vi "Unreserve(Session).vi"(8 "error in (no error)":errorcluster, 9 "InstrumentHandle_port in":u32[](array[numeric]), 10 "InstrumentHandle_board in":u32[](array[numeric])) -> (0 "error out":errorcluster)   [LabVIEW 2020, in "AIM664LV.lvlib"]
uses:
  AIM664LV.lvlib
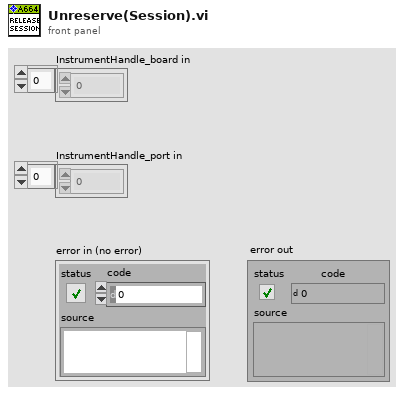
[diagram p1: front panel]
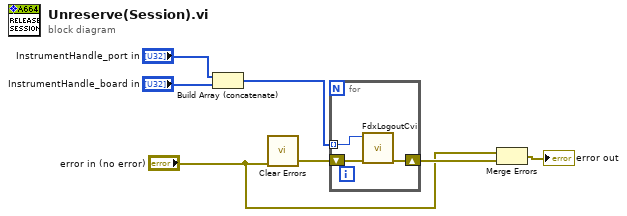
[diagram p0: block diagram]
diagram:
  n1 = Build Array (concatenate)("InstrumentHandle_port in", "InstrumentHandle_board in") -> (w1:u32[])
  n2 = call <vilib>:"Clear Errors.vi"("error in (no error)"="error in (no error)") -> ("error out"=w7:errorcluster)  [unwired: 5 in, 1 out]
  n3 = for {
    shift-right: [w9] -> w6
    shift-left: w7 -> [w10]
    tunnel: w1 -> [w8] mode=indexing
    n4 = call "FdxLogoutCvi.vi"("error in"=w10, "InstrumentHandle"=w8) -> ("error out"=w9:errorcluster)  [unwired: 9 in]
  }
  n5 = Merge Errors("error in (no error)", w6) -> (→"error out":errorcluster)
